vi "LJM_eWriteAddress.vi"(0 "Handle In":i32, 5 "Address":i32, 7 "Type":i32, 9 "Value":dbl format="%.2f", 11 "error in":errorcluster) -> (4 "Handle Out":i32, 15 "error out":errorcluster)   [LabVIEW 2020]
uses:
  Library/Frameworks/LabJackM.framework
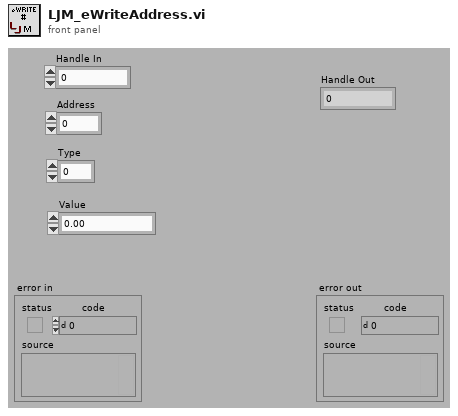
[diagram p1: front panel]
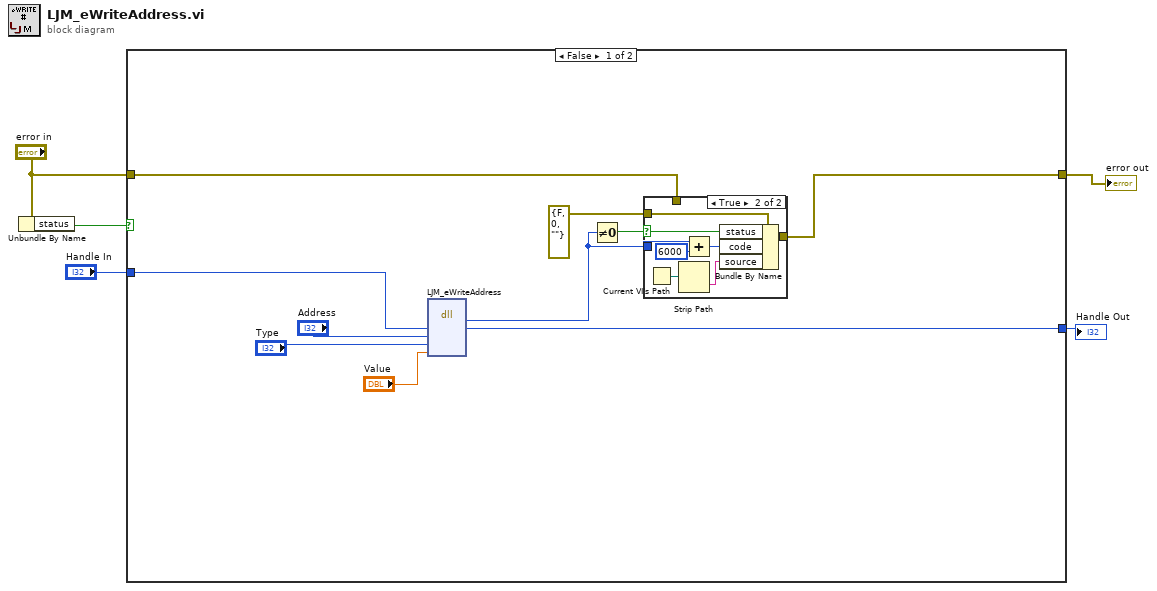
[diagram p0: block diagram]
diagram:
  n1 = Unbundle By Name("error in") -> ("status"=w5:bool)
  n2 = case shown="False" w5 {
    tunnel: "error in" -> [w12 w26]
    tunnel: [w11 w26] -> w3
    tunnel: "Handle In" -> [w7 w25]
    tunnel: [w6 w25] -> w1
    frame False {
      n3 = dll-call lib="Library/Frameworks/LabJackM.framework" fn="LJM_eWriteAddress"("Handle"=w7, "Address"="Address", "Type"="Type", "Value"="Value") -> ("return type"=w15:i32, "Handle"=w6:i32)  [unwired: 6 in, 2 out]
      n4 = Not Equal To 0?(x=w15) -> (x != 0?=w14:bool)
      n5 = case shown="True" w14 {
        selector: w14 -> [_ w23]
        tunnel: [w16 w24] -> w11
        tunnel: errorcluster {"status"=FALSE, "code"=0, "source"=""} ("error IO") -> [_ w22]
        tunnel: w15 -> [_ w18]
        tunnel: w12 -> [w16 _]
        frame False {
        }
        frame True {
          n6 = Current VI's Path() -> (path=w20:path)
          n7 = Strip Path(path=w20) -> (name=w21:string)  [unwired: 1 out]
          n8 = Add(x=w18, y=6000) -> (x+y=w19:i32)
          n9 = Bundle By Name(cluster=w22, "status"=w23, "code"=w19, "source"=w21) -> (w24:errorcluster)
        }
      }
    }
    frame True {
    }
  }
  "error out" <- w3
  "Handle Out" <- w1
